vi "Compile Resistor.vi"(8 "error in (no error)":errorcluster, 11 "Device Item Ref in":T5 format="%.0x") -> (0 "error out":errorcluster, 1 "Resistor Engine Data":T1 {"Ordered Channels" format="%.0x"; "RT IDs"."Slot #" max=15; "RT IDs"."Chip Address (A2 A1 A0)" max=7}, 2 "Initial Resistor SPI CMDs":u64[](array[numeric]), 3 "Device Item Ref out":T5 format="%.0x")   [LabVIEW 2014, in "SLSC configuration System Explorer.lvlib"]
uses:
  SLSC configuration System Explorer.lvlib
  <vilib>/NI Veristand/Custom Device API/Custom Device Item Ref.ctl
  Shared/Type Defs/RT Engine Data.ctl
  Shared/Type Defs/RT IDs.ctl
  Shared/SPI Utility/Slot #.ctl
  Shared/MCP23S17/Chip Address.ctl
  Shared/Constants.vi
  <vilib>/NI Veristand/Custom Device Tools/Custom Device Utility Library/Custom Device Utility Library.lvlib
  Shared/SLSC configuration Shared.lvlib
  <vilib>/NI Veristand/Custom Device API/Custom Device API.lvlib
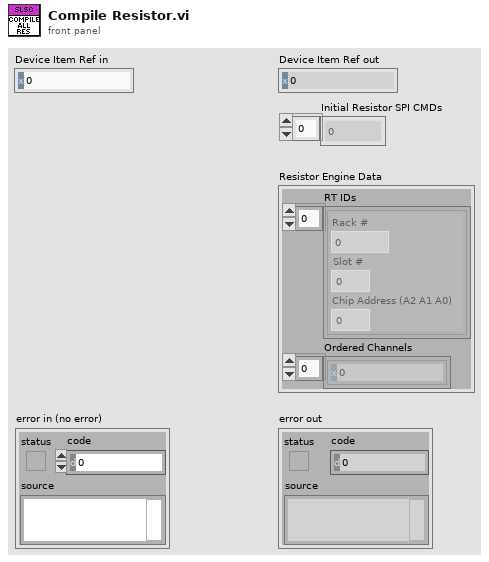
[diagram p1: front panel]
types:
  T1 = typedef "SLSC configuration Shared.lvlib/RT Engine Data.ctl" = cluster{"RT IDs":T2[], "Ordered Channels":T5[]}
  T2 = typedef "SLSC configuration Shared.lvlib/RT IDs.ctl" = cluster{"Rack #":u8, "Slot #":T3, "Chip Address (A2 A1 A0)":T4}
  T3 = typedef "SLSC configuration Shared.lvlib/Slot #.ctl" = u8
  T4 = typedef "SLSC configuration Shared.lvlib/Chip Address.ctl" = u8
  T5 = typedef "Custom Device API.lvlib/Custom Device Item Ref.ctl" = u64
  T6 = typedef "SLSC configuration Shared.lvlib/Card Position.ctl" = cluster{"Rack #":u8, "Slot #":T3}
  T7 = typedef "SLSC configuration Shared.lvlib/Resistance.ctl" = dbl
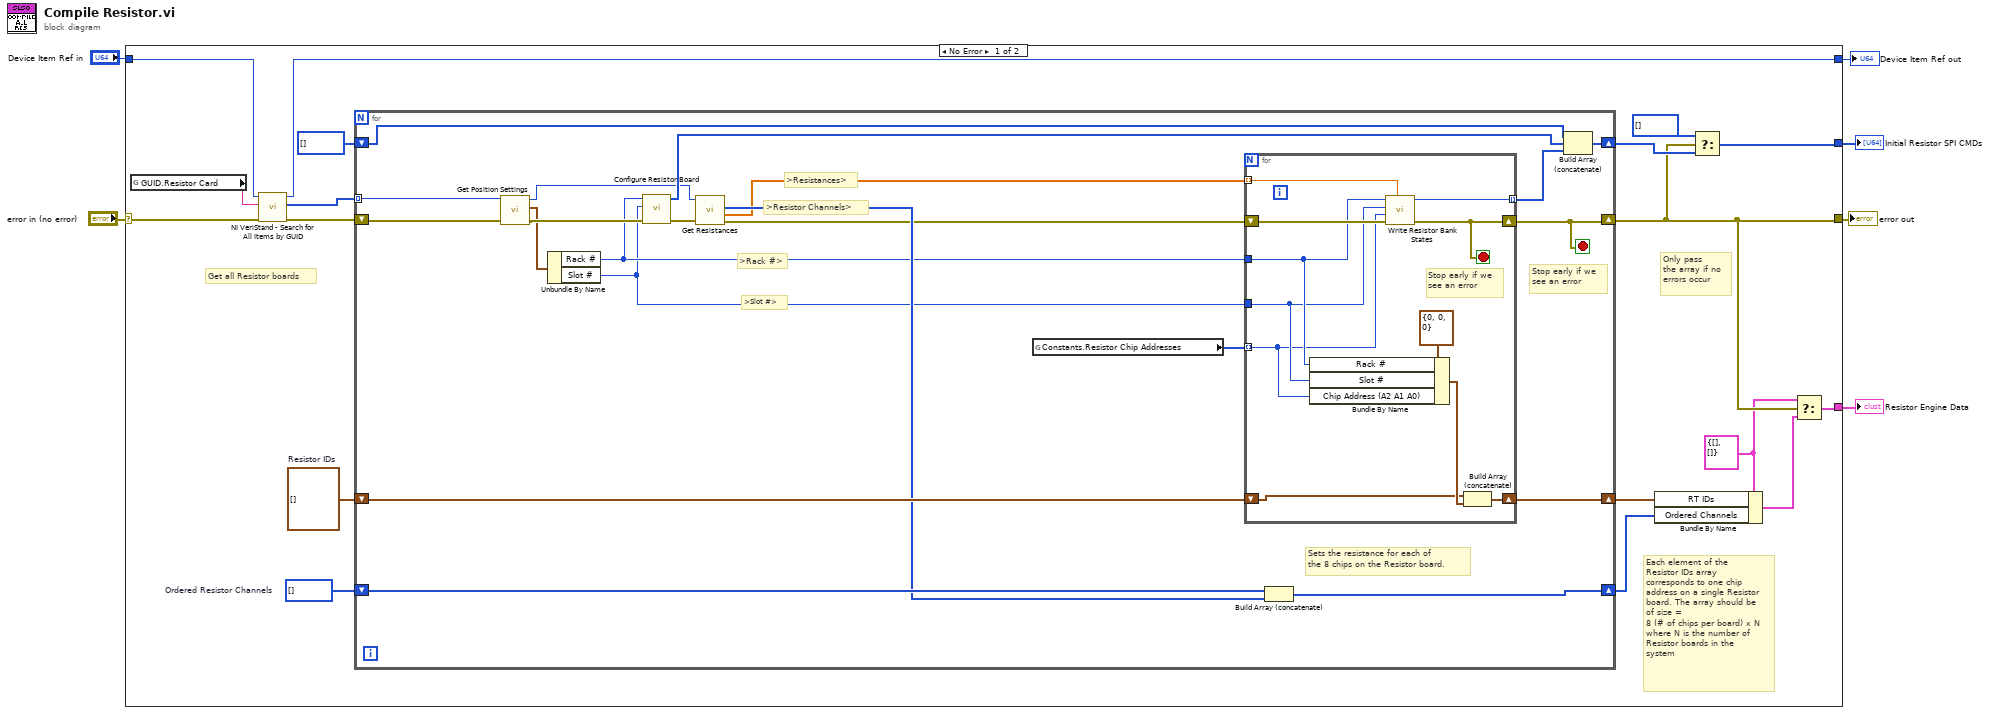
[diagram p0: block diagram]
diagram:
  n1 = case shown="No Error" "error in (no error)" {
    selector: "error in (no error)" -> [w21 w58]
    tunnel: [w10 w58] -> w6
    tunnel: "Device Item Ref in" -> [w15 w57]
    tunnel: [w7 _] -> w3
    tunnel: [w11 _] -> w2
    tunnel: [w14 w57] -> w1
    frame No Error {
      w9 = T1 {"RT IDs"=[], "Ordered Channels"=[]} ("FIU Engine Data")
      w18 = T5[] []  # Ordered Resistor Channels
      w19 = T2[] []  # Resistor IDs
      # "Only pass\nthe array if no\nerrors occur"
      # "Get all Resistor boards"
      # "Each element of the Resistor IDs array corresponds to one chip address on a single Resistor board. The array should be of size =\n8 (# of chips per board) x N where N is the number of Resistor boards in the system"
      n2 = global read "Constants.vi" "GUID.Resistor Card"() -> (w24:string)
      n3 = call <vilib>:"NI VeriStand - Search for All Items by GUID.vi"("error in"=w21, "Item GUID"=w24, "Section Ref in"=w15) -> ("error out"=w23:errorcluster, "Item Refs"=w22:T5[], "Section Ref out"=w14:T5)  [unwired: 5 in, 1 out]
      n4 = for {
        tunnel: w22 -> [w31] mode=indexing
        shift-right: [w34] -> w10
        shift-left: w23 -> [w32]
        shift-right: [w41] -> w13
        shift-left: u64[] [] ("SPI FIFO Messages") -> [w45]
        shift-right: [w39] -> w17
        shift-left: w19 -> [w40]
        shift-right: [w37] -> w16
        shift-left: w18 -> [w38]
        stop <- w34 stop-if-true
        # "Stop early if we\nsee an error"
        # ">Resistances>"
        # ">Resistor Channels>"
        # "Sets the resistance for each of\nthe 8 chips on the Resistor board."
        # ">Slot #>"
        # ">Rack #>"
        n5 = call "Get Position Settings.vi"("error in (no error)"=w32, "Item Ref in"=w31) -> ("error out"=w29:errorcluster, "Card Position"=w28:T6, "Item Ref out"=w30:T5)  [unwired: 7 in]
        n6 = Unbundle By Name(w28) -> ("Rack #"=w27:u8, "Slot #"=w26:T3)
        n7 = call "Configure Resistor Board.vi"("error in (no error)"=w29, "Slot #"=w26, "Rack #"=w27) -> ("error out"=w43:errorcluster, "SPI FIFO Messages"=w44:u64[])  [unwired: 7 in]
        n8 = call "Get Resistances.vi"("error in (no error)"=w43, "Item Ref in"=w30) -> ("error out"=w35:errorcluster, "Resistor Resistances"=w25:T7[], "Ordered Resistor Channels"=w36:T5[])  [unwired: 6 in, 1 out]
        n9 = global read "Constants.vi" "Constants.Resistor Chip Addresses"() -> (w33:u8[])
        n10 = for {
          tunnel: w33 -> [w51] mode=indexing
          shift-right: [w46] -> w34
          shift-left: w35 -> [w56]
          tunnel: w26 -> [w52]
          tunnel: w27 -> [w53]
          tunnel: [w55] -> w42 mode=indexing
          shift-right: [w48] -> w39
          shift-left: w40 -> [w49]
          tunnel: w25 -> [w47] mode=indexing
          stop <- w46 stop-if-true
          # "Stop early if we\nsee an error"
          n11 = Bundle By Name(cluster=T2 {"Rack #"=0, "Slot #"=0, "Chip Address (A2 A1 A0)"=0}, "Rack #"=w53, "Slot #"=w52, "Chip Address (A2 A1 A0)"=w51) -> (w50:T2)
          n12 = call "Write Resistor Bank States.vi"("Output Cache in"=w47, "error in (no error)"=w56, "Chip Address (A2 A1 A0)"=w51, "Slot #"=w52, "Rack #"=w53) -> ("error out"=w46:errorcluster, "FIFO SPI Message"=w55:u64)  [unwired: 4 in, 1 out]
          n13 = Build Array (concatenate)(w49, w50) -> (w48:T2[])
        }
        n14 = Build Array (concatenate)(w38, w36) -> (w37:T5[])
        n15 = Build Array (concatenate)(w45, w44, w42) -> (w41:u64[])
      }
      n16 = Bundle By Name(cluster=w9, "RT IDs"=w17, "Ordered Channels"=w16) -> (w8:T1)
      n17 = Select(t=u64[] [], s=w10, f=w13) -> (s? t:f=w11:u64[])
      n18 = Select(t=w9, s=w10, f=w8) -> (s? t:f=w7:T1)
    }
    frame Error {
    }
  }
  "error out" <- w6
  "Device Item Ref out" <- w1
  "Resistor Engine Data" <- w3
  "Initial Resistor SPI CMDs" <- w2
